vi "Test Coffee Shop List Cashiers.vi"(8 "error in (no error)":errorcluster, 11 "Coffee Shop Test In":refnum<class "Coffee Shop Test.lvclass">) -> (0 "error out":errorcluster, 3 "Coffee Shop Test Out":refnum<class "Coffee Shop Test.lvclass">)   [LabVIEW 2020, in "Coffee Shop Test.lvclass"]
uses:
  Coffee Shop Test.lvclass
  C:/Program Files (x86)/National Instruments/LabVIEW 2020/vi.lib/Asteme/LUnit/Test Case.lvclass
  Coffee Shop/Coffee Shop.lvclass
  C:/Program Files (x86)/National Instruments/LabVIEW 2020/vi.lib/Asteme/Triarc Framework/Process/Process.lvclass
  <vilib>/Asteme/Triarc Framework/Process/Process.lvclass/Process.ctl
  <vilib>/Asteme/LUnit/Test Case.lvclass/Test Case.ctl
  <vilib>/Asteme/LUnit/LUnit Assertion Result.lvclass/LUnit Assertion Result.ctl
  <vilib>/Asteme/Triarc Framework/Process/Private/SubVIs/Wait for finish.vi
  <vilib>/Asteme/Triarc Framework/Process/Protected/Messaging/Enqueue Message.vi
  <vilib>/Asteme/Triarc Framework/Process/Private/SubVIs/Set Lifecycle State.vi
  <vilib>/Asteme/Triarc Framework/Process/Public/Lifecycle/Get Lifecycle State.vi
  <vilib>/Asteme/LUnit/Palette/Pass.vi
  <vilib>/Asteme/LUnit/Palette/Fail.vi
  <vilib>/Asteme/LUnit/Variant to string.vi
  <vilib>/Asteme/LUnit/Set Assertion Type.vi
  <vilib>/AdvancedString/1D String Array to Delimited String.vi
  <vilib>/Utility/error.llb/Clear Errors.vi
  <vilib>/Asteme/LUnit/Add test result.vi
  <vilib>/Asteme/LUnit/LUnit Write Passed.vi
  <vilib>/Asteme/LUnit/LUnit Get Test Case.vi
  <vilib>/Asteme/LUnit/Assertion Result/LUnit Get Test Name.vi
  <vilib>/Asteme/LUnit/LUnit Write Message.vi
  <vilib>/Asteme/LUnit/LUnit Write Description.vi
  <vilib>/Asteme/LUnit/LUnit Write Assertion Type.vi
  <vilib>/Asteme/LUnit/Read Test Case Name.vi
  <vilib>/Utility/error.llb/Error Cluster From Error Code.vi
  <vilib>/Utility/Data Type/Get Type Information.vi
  <vilib>/Utility/LVClass/Get LV Class Name.vi
  <vilib>/Asteme/LUnit/LUnit Assertion Result.lvclass
  <vilib>/Asteme/Triarc Framework/Process/Process.lvclass
  <vilib>/Asteme/LUnit/Test Case.lvclass
  C:/Program Files (x86)/National Instruments/LabVIEW 2020/vi.lib/Asteme/Triarc Framework/Application/Application.lvclass
  C:/Program Files (x86)/National Instruments/LabVIEW 2020/vi.lib/Asteme/Triarc Framework/Base/Base.lvclass
  C:/Program Files (x86)/National Instruments/LabVIEW 2020/vi.lib/Asteme/Triarc Framework/Error Handler Interface/Error Handler Interface.lvclass
  C:/Program Files (x86)/National Instruments/LabVIEW 2020/vi.lib/Asteme/Triarc Framework/Logging/Logging.lvclass
  C:/Users/anton/Documents/GitHub/Triarc-Examples/Coffee Shop/Coffee Shop/Coffee Shop.lvclass
  C:/Program Files (x86)/National Instruments/LabVIEW 2020/vi.lib/Asteme/Triarc Framework Test Suite/Application Test/Application Test.lvclass
  C:/Program Files (x86)/National Instruments/LabVIEW 2020/vi.lib/Asteme/Triarc Framework Test Suite/Process Test/Process Test.lvclass
  C:/Program Files (x86)/National Instruments/LabVIEW 2020/vi.lib/Asteme/Triarc Framework Test Suite/Base Class Test/Base Test.lvclass
  C:/Users/anton/Documents/GitHub/Triarc-Examples/Coffee Shop/Coffee Shop Test/Coffee Shop Test.lvclass
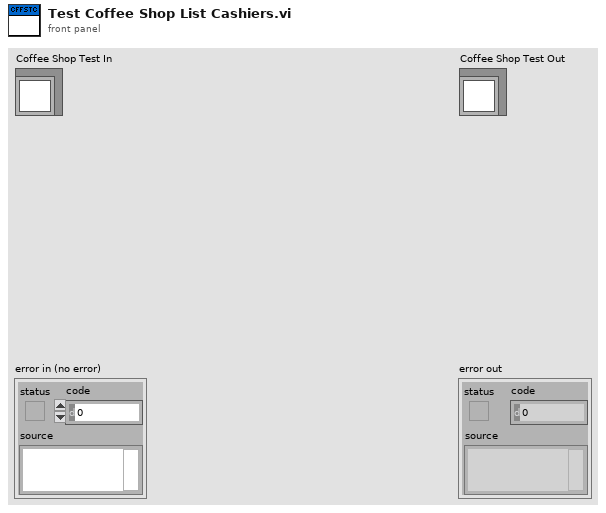
[diagram p1: front panel]
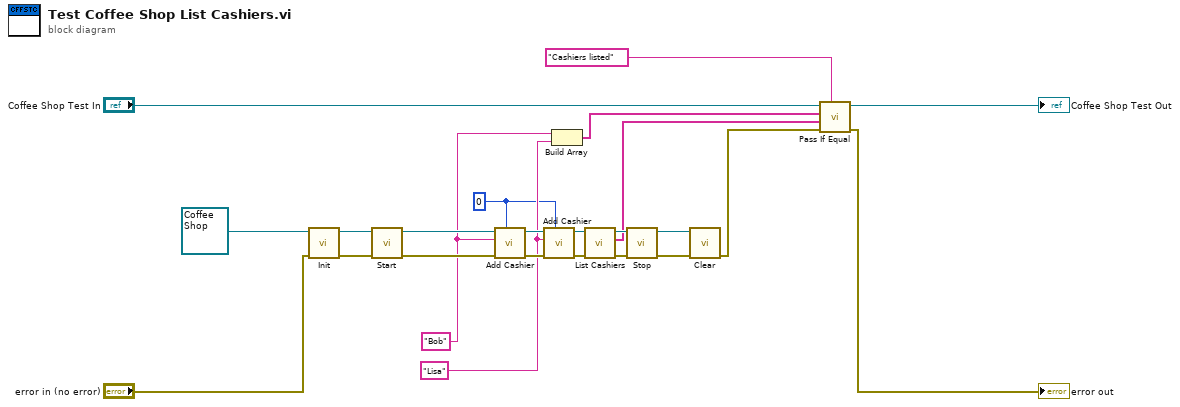
[diagram p0: block diagram]
diagram:
  w1 = u32 0 ("Time Scale [ms]")
  w4 = "Lisa"
  w5 = "Bob" ("Name")
  n1 = call-dynamic "Init.vi"("error in (no error)"="error in (no error)", "Process In"=refnum<class "Coffee Shop.lvclass"> refnum ("Coffee Shop.lvclass")) -> ("error out"=w22:errorcluster, "Process Out"=w23:refnum<class "Coffee Shop.lvclass">)  [unwired: 8 in]
  n2 = call <vilib>:"Start.vi"("error in (no error)"=w22, "Process In"=w23) -> ("error out"=w17:errorcluster, "Process Out"=w16:refnum<class "Coffee Shop.lvclass">)  [unwired: 8 in]
  n3 = call "Add Cashier.vi"("Time Scale [ms]"=w1, "error in (no error)"=w17, "Name"=w5, "Coffee Shop in"=w16) -> ("error out"=w18:errorcluster, "Coffee Shop out"=w9:refnum<class "Coffee Shop.lvclass">)  [unwired: 6 in]
  n4 = call "Add Cashier.vi"("Time Scale [ms]"=w1, "error in (no error)"=w18, "Name"=w4, "Coffee Shop in"=w9) -> ("error out"=w10:errorcluster, "Coffee Shop out"=w7:refnum<class "Coffee Shop.lvclass">)  [unwired: 6 in]
  n5 = Build Array(w5, w4) -> (w3:string[])
  n6 = call "List Cashiers.vi"("error in (no error)"=w10, "Coffee Shop in"=w7) -> ("error out"=w8:errorcluster, "Names"=w2:string[], "Coffee Shop out"=w6:refnum<class "Coffee Shop.lvclass">)  [unwired: 7 in]
  n7 = call <vilib>:"Stop.vi"("error in (no error)"=w8, "Process In"=w6) -> ("error out"=w20:errorcluster, "Process Out"=w21:refnum<class "Coffee Shop.lvclass">)  [unwired: 7 in, 1 out]
  n8 = call-dynamic "Clear.vi"("error in (no error)"=w20, "Application In"=w21) -> ("error out"=w13:errorcluster)  [unwired: 9 in]
  n9 = call <vilib>:"Pass If Equal.vi"("Description"="Cashiers listed", "error in (no error)"=w13, "Actual"=w2, "Expected"=w3, "Test Case In"="Coffee Shop Test In") -> ("error out"=→"error out":errorcluster, "Test Case Out"=→"Coffee Shop Test Out":refnum<class "Coffee Shop Test.lvclass">)  [unwired: 5 in]
